vi "Read Settings File.vi"(8 "error in":errorcluster, 11 "Cluster in":T1 {"Gain Array"."Gain 17" format="%.2f"; "Gain Array"."Gain 16" format="%.2f"; "Gain Array"."Gain 15" format="%.2f"; "Gain Array"."Gain 14" format="%.2f"; "Gain Array"."Gain 13" format="%.2f"; "Gain Array"."Gain 12" format="%.2f"; "Gain Array"."Gain 11" format="%.2f"; "Gain Array"."Gain 10" format="%.2f"; "Gain Array"."Gain 9" format="%.2f"; "Gain Array"."Gain 8" format="%.2f"; "Gain Array"."Gain 7" format="%.2f"; "Gain Array"."Gain 6" format="%.2f"; "Gain Array"."Gain 5" format="%.2f"; "Gain Array"."Gain 4" format="%.2f"; "Gain Array"."Gain 3" format="%.2f"; "Gain Array"."Gain 2" format="%.2f"; "Gain Array"."Gain 1" format="%.2f"; "Gains"."Gain 6" format="%.2f"; "Gains"."Gain 5" format="%.2f"; "Gains"."Gain 4" format="%.2f"; "Gains"."Gain 3" format="%.2f"; "Gains"."Gain 2" format="%.2f"; "Gains"."Gain 1" format="%.2f"; "User Gains"."Gain 6" format="%.2f"; "User Gains"."Gain 5" format="%.2f"; "User Gains"."Gain 4" format="%.2f"; "User Gains"."Gain 3" format="%.2f"; "User Gains"."Gain 2" format="%.2f"; "User Gains"."Gain 1" format="%.2f"; "Channel Configuration List"."Channel Configuration Cluster 17"."Current Range" items=["1 <500m>"=0.5, "2 <1>"=1.0, "5 <2.5>"=2.5, "10 <5>"=5.0, "20 <10>"=10.0, "50 <25>"=25.0]; "Channel Configuration List"."Channel Configuration Cluster 17"."Voltage Range" items=["1.5 <0.75>"=0.75, "3 <1.5>"=1.5, "6 <3>"=3.0, "10 <5>"=5.0, "15 <7.5>"=7.5, "30 <15>"=15.0, "60 <30>"=30.0, "100 <50>"=50.0, "150 <75>"=75.0, "300 <150>"=150.0, "600 <300>"=300.0, "1000 <500>"=500.0]; "Channel Configuration List"."Channel Configuration Cluster 16"."Current Range" items=["1 <500m>"=0.5, "2 <1>"=1.0, "5 <2.5>"=2.5, "10 <5>"=5.0, "20 <10>"=10.0, "50 <25>"=25.0]; "Channel Configuration List"."Channel Configuration Cluster 16"."Voltage Range" items=["1.5 <0.75>"=0.75, "3 <1.5>"=1.5, "6 <3>"=3.0, "10 <5>"=5.0, "15 <7.5>"=7.5, "30 <15>"=15.0, "60 <30>"=30.0, "100 <50>"=50.0, "150 <75>"=75.0, "300 <150>"=150.0, "600 <300>"=300.0, "1000 <500>"=500.0]; "Channel Configuration List"."Channel Configuration Cluster 15"."Current Range" items=["1 <500m>"=0.5, "2 <1>"=1.0, "5 <2.5>"=2.5, "10 <5>"=5.0, "20 <10>"=10.0, "50 <25>"=25.0]; "Channel Configuration List"."Channel Configuration Cluster 15"."Voltage Range" items=["1.5 <0.75>"=0.75, "3 <1.5>"=1.5, "6 <3>"=3.0, "10 <5>"=5.0, "15 <7.5>"=7.5, "30 <15>"=15.0, "60 <30>"=30.0, "100 <50>"=50.0, "150 <75>"=75.0, "300 <150>"=150.0, "600 <300>"=300.0, "1000 <500>"=500.0]; "Channel Configuration List"."Channel Configuration Cluster 14"."Current Range" items=["1 <500m>"=0.5, "2 <1>"=1.0, "5 <2.5>"=2.5, "10 <5>"=5.0, "20 <10>"=10.0, "50 <25>"=25.0]; "Channel Configuration List"."Channel Configuration Cluster 14"."Voltage Range" items=["1.5 <0.75>"=0.75, "3 <1.5>"=1.5, "6 <3>"=3.0, "10 <5>"=5.0, "15 <7.5>"=7.5, "30 <15>"=15.0, "60 <30>"=30.0, "100 <50>"=50.0, "150 <75>"=75.0, "300 <150>"=150.0, "600 <300>"=300.0, "1000 <500>"=500.0]; "Channel Configuration List"."Channel Configuration Cluster 13"."Current Range" items=["1 <500m>"=0.5, "2 <1>"=1.0, "5 <2.5>"=2.5, "10 <5>"=5.0, "20 <10>"=10.0, "50 <25>"=25.0]; "Channel Configuration List"."Channel Configuration Cluster 13"."Voltage Range" items=["1.5 <0.75>"=0.75, "3 <1.5>"=1.5, "6 <3>"=3.0, "10 <5>"=5.0, "15 <7.5>"=7.5, "30 <15>"=15.0, "60 <30>"=30.0, "100 <50>"=50.0, "150 <75>"=75.0, "300 <150>"=150.0, "600 <300>"=300.0, "1000 <500>"=500.0]; "Channel Configuration List"."Channel Configuration Cluster 12"."Current Range" items=["1 <500m>"=0.5, "2 <1>"=1.0, "5 <2.5>"=2.5, "10 <5>"=5.0, "20 <10>"=10.0, "50 <25>"=25.0]; "Channel Configuration List"."Channel Configuration Cluster 12"."Voltage Range" items=["1.5 <0.75>"=0.75, "3 <1.5>"=1.5, "6 <3>"=3.0, "10 <5>"=5.0, "15 <7.5>"=7.5, "30 <15>"=15.0, "60 <30>"=30.0, "100 <50>"=50.0, "150 <75>"=75.0, "300 <150>"=150.0, "600 <300>"=300.0, "1000 <500>"=500.0]; "Channel Configuration List"."Channel Configuration Cluster 11"."Current Range" items=["1 <500m>"=0.5, "2 <1>"=1.0, "5 <2.5>"=2.5, "10 <5>"=5.0, "20 <10>"=10.0, "50 <25>"=25.0]; "Channel Configuration List"."Channel Configuration Cluster 11"."Voltage Range" items=["1.5 <0.75>"=0.75, "3 <1.5>"=1.5, "6 <3>"=3.0, "10 <5>"=5.0, "15 <7.5>"=7.5, "30 <15>"=15.0, "60 <30>"=30.0, "100 <50>"=50.0, "150 <75>"=75.0, "300 <150>"=150.0, "600 <300>"=300.0, "1000 <500>"=500.0]; "Channel Configuration List"."Channel Configuration Cluster 10"."Current Range" items=["1 <500m>"=0.5, "2 <1>"=1.0, "5 <2.5>"=2.5, "10 <5>"=5.0, "20 <10>"=10.0, "50 <25>"=25.0]; "Channel Configuration List"."Channel Configuration Cluster 10"."Voltage Range" items=["1.5 <0.75>"=0.75, "3 <1.5>"=1.5, "6 <3>"=3.0, "10 <5>"=5.0, "15 <7.5>"=7.5, "30 <15>"=15.0, "60 <30>"=30.0, "100 <50>"=50.0, "150 <75>"=75.0, "300 <150>"=150.0, "600 <300>"=300.0, "1000 <500>"=500.0]; "Channel Configuration List"."Channel Configuration Cluster 9"."Voltage Range" items=["1.5 <0.75>"=0.75, "3 <1.5>"=1.5, "6 <3>"=3.0, "10 <5>"=5.0, "15 <7.5>"=7.5, "30 <15>"=15.0, "60 <30>"=30.0, "100 <50>"=50.0, "150 <75>"=75.0, "300 <150>"=150.0, "600 <300>"=300.0, "1000 <500>"=500.0]; "Channel Configuration List"."Channel Configuration Cluster 9"."Current Range" items=["10m <5m>"=0.005, "20m <10m>"=0.01, "50m <25m>"=0.025, "100m <50m>"=0.05, "200m <100m>"=0.1, "500m <250m>"=0.25, "1 <500m>"=0.5, "2 <1>"=1.0, "5 <2.5>"=2.5]; "Channel Configuration List"."Channel Configuration Cluster 8"."Voltage Range" items=["1.5 <0.75>"=0.75, "3 <1.5>"=1.5, "6 <3>"=3.0, "10 <5>"=5.0, "15 <7.5>"=7.5, "30 <15>"=15.0, "60 <30>"=30.0, "100 <50>"=50.0, "150 <75>"=75.0, "300 <150>"=150.0, "600 <300>"=300.0, "1000 <500>"=500.0]; "Channel Configuration List"."Channel Configuration Cluster 8"."Current Range" items=["10m <5m>"=0.005, "20m <10m>"=0.01, "50m <25m>"=0.025, "100m <50m>"=0.05, "200m <100m>"=0.1, "500m <250m>"=0.25, "1 <500m>"=0.5, "2 <1>"=1.0, "5 <2.5>"=2.5]; "Channel Configuration List"."Channel Configuration Cluster 7"."Voltage Range" items=["1.5 <0.75>"=0.75, "3 <1.5>"=1.5, "6 <3>"=3.0, "10 <5>"=5.0, "15 <7.5>"=7.5, "30 <15>"=15.0, "60 <30>"=30.0, "100 <50>"=50.0, "150 <75>"=75.0, "300 <150>"=150.0, "600 <300>"=300.0, "1000 <500>"=500.0]; "Channel Configuration List"."Channel Configuration Cluster 7"."Current Range" items=["10m <5m>"=0.005, "20m <10m>"=0.01, "50m <25m>"=0.025, "100m <50m>"=0.05, "200m <100m>"=0.1, "500m <250m>"=0.25, "1 <500m>"=0.5, "2 <1>"=1.0, "5 <2.5>"=2.5]; "Channel Configuration List"."Channel Configuration Cluster 6"."Voltage Range" items=["1.5 <0.75>"=0.75, "3 <1.5>"=1.5, "6 <3>"=3.0, "10 <5>"=5.0, "15 <7.5>"=7.5, "30 <15>"=15.0, "60 <30>"=30.0, "100 <50>"=50.0, "150 <75>"=75.0, "300 <150>"=150.0, "600 <300>"=300.0, "1000 <500>"=500.0]; "Channel Configuration List"."Channel Configuration Cluster 6"."Current Range" items=["10m <5m>"=0.005, "20m <10m>"=0.01, "50m <25m>"=0.025, "100m <50m>"=0.05, "200m <100m>"=0.1, "500m <250m>"=0.25, "1 <500m>"=0.5, "2 <1>"=1.0, "5 <2.5>"=2.5]; "Channel Configuration List"."Channel Configuration Cluster 5"."Voltage Range" items=["1.5 <0.75>"=0.75, "3 <1.5>"=1.5, "6 <3>"=3.0, "10 <5>"=5.0, "15 <7.5>"=7.5, "30 <15>"=15.0, "60 <30>"=30.0, "100 <50>"=50.0, "150 <75>"=75.0, "300 <150>"=150.0, "600 <300>"=300.0, "1000 <500>"=500.0]; "Channel Configuration List"."Channel Configuration Cluster 5"."Current Range" items=["10m <5m>"=0.005, "20m <10m>"=0.01, "50m <25m>"=0.025, "100m <50m>"=0.05, "200m <100m>"=0.1, "500m <250m>"=0.25, "1 <500m>"=0.5, "2 <1>"=1.0, "5 <2.5>"=2.5]; "Channel Configuration List"."Channel Configuration Cluster 4"."Voltage Range" items=["1.5 <0.75>"=0.75, "3 <1.5>"=1.5, "6 <3>"=3.0, "10 <5>"=5.0, "15 <7.5>"=7.5, "30 <15>"=15.0, "60 <30>"=30.0, "100 <50>"=50.0, "150 <75>"=75.0, "300 <150>"=150.0, "600 <300>"=300.0, "1000 <500>"=500.0]; "Channel Configuration List"."Channel Configuration Cluster 4"."Current Range" items=["10m <5m>"=0.005, "20m <10m>"=0.01, "50m <25m>"=0.025, "100m <50m>"=0.05, "200m <100m>"=0.1, "500m <250m>"=0.25, "1 <500m>"=0.5, "2 <1>"=1.0, "5 <2.5>"=2.5]; "Channel Configuration List"."Channel Configuration Cluster 3"."Voltage Range" items=["1.5 <0.75>"=0.75, "3 <1.5>"=1.5, "6 <3>"=3.0, "10 <5>"=5.0, "15 <7.5>"=7.5, "30 <15>"=15.0, "60 <30>"=30.0, "100 <50>"=50.0, "150 <75>"=75.0, "300 <150>"=150.0, "600 <300>"=300.0, "1000 <500>"=500.0]; "Channel Configuration List"."Channel Configuration Cluster 3"."Current Range" items=["10m <5m>"=0.005, "20m <10m>"=0.01, "50m <25m>"=0.025, "100m <50m>"=0.05, "200m <100m>"=0.1, "500m <250m>"=0.25, "1 <500m>"=0.5, "2 <1>"=1.0, "5 <2.5>"=2.5]; "Channel Configuration List"."Channel Configuration Cluster 2"."Voltage Range" items=["1.5 <0.75>"=0.75, "3 <1.5>"=1.5, "6 <3>"=3.0, "10 <5>"=5.0, "15 <7.5>"=7.5, "30 <15>"=15.0, "60 <30>"=30.0, "100 <50>"=50.0, "150 <75>"=75.0, "300 <150>"=150.0, "600 <300>"=300.0, "1000 <500>"=500.0]; "Channel Configuration List"."Channel Configuration Cluster 2"."Current Range" items=["10m <5m>"=0.005, "20m <10m>"=0.01, "50m <25m>"=0.025, "100m <50m>"=0.05, "200m <100m>"=0.1, "500m <250m>"=0.25, "1 <500m>"=0.5, "2 <1>"=1.0, "5 <2.5>"=2.5]; "Channel Configuration List"."Channel Configuration Cluster"."Voltage Range" items=["1.5 <0.75>"=0.75, "3 <1.5>"=1.5, "6 <3>"=3.0, "10 <5>"=5.0, "15 <7.5>"=7.5, "30 <15>"=15.0, "60 <30>"=30.0, "100 <50>"=50.0, "150 <75>"=75.0, "300 <150>"=150.0, "600 <300>"=300.0, "1000 <500>"=500.0]; "Channel Configuration List"."Channel Configuration Cluster"."Current Range" items=["10m <5m>"=0.005, "20m <10m>"=0.01, "50m <25m>"=0.025, "100m <50m>"=0.05, "200m <100m>"=0.1, "500m <250m>"=0.25, "1 <500m>"=0.5, "2 <1>"=1.0, "5 <2.5>"=2.5]; "Settling Delay" min=0.0 format="%<%H:%M:%S>t"}) -> (0 "error out":errorcluster, 2 "status":bool, 3 "Cluster out":T1 {"Gain Array"."Gain 17" format="%.2f"; "Gain Array"."Gain 16" format="%.2f"; "Gain Array"."Gain 15" format="%.2f"; "Gain Array"."Gain 14" format="%.2f"; "Gain Array"."Gain 13" format="%.2f"; "Gain Array"."Gain 12" format="%.2f"; "Gain Array"."Gain 11" format="%.2f"; "Gain Array"."Gain 10" format="%.2f"; "Gain Array"."Gain 9" format="%.2f"; "Gain Array"."Gain 8" format="%.2f"; "Gain Array"."Gain 7" format="%.2f"; "Gain Array"."Gain 6" format="%.2f"; "Gain Array"."Gain 5" format="%.2f"; "Gain Array"."Gain 4" format="%.2f"; "Gain Array"."Gain 3" format="%.2f"; "Gain Array"."Gain 2" format="%.2f"; "Gain Array"."Gain 1" format="%.2f"; "Gains"."Gain 6" format="%.2f"; "Gains"."Gain 5" format="%.2f"; "Gains"."Gain 4" format="%.2f"; "Gains"."Gain 3" format="%.2f"; "Gains"."Gain 2" format="%.2f"; "Gains"."Gain 1" format="%.2f"; "User Gains"."Gain 6" format="%.2f"; "User Gains"."Gain 5" format="%.2f"; "User Gains"."Gain 4" format="%.2f"; "User Gains"."Gain 3" format="%.2f"; "User Gains"."Gain 2" format="%.2f"; "User Gains"."Gain 1" format="%.2f"; "Channel Configuration List"."Channel Configuration Cluster 17"."Current Range" items=["1 <500m>"=0.5, "2 <1>"=1.0, "5 <2.5>"=2.5, "10 <5>"=5.0, "20 <10>"=10.0, "50 <25>"=25.0]; "Channel Configuration List"."Channel Configuration Cluster 17"."Voltage Range" items=["1.5 <0.75>"=0.75, "3 <1.5>"=1.5, "6 <3>"=3.0, "10 <5>"=5.0, "15 <7.5>"=7.5, "30 <15>"=15.0, "60 <30>"=30.0, "100 <50>"=50.0, "150 <75>"=75.0, "300 <150>"=150.0, "600 <300>"=300.0, "1000 <500>"=500.0]; "Channel Configuration List"."Channel Configuration Cluster 16"."Current Range" items=["1 <500m>"=0.5, "2 <1>"=1.0, "5 <2.5>"=2.5, "10 <5>"=5.0, "20 <10>"=10.0, "50 <25>"=25.0]; "Channel Configuration List"."Channel Configuration Cluster 16"."Voltage Range" items=["1.5 <0.75>"=0.75, "3 <1.5>"=1.5, "6 <3>"=3.0, "10 <5>"=5.0, "15 <7.5>"=7.5, "30 <15>"=15.0, "60 <30>"=30.0, "100 <50>"=50.0, "150 <75>"=75.0, "300 <150>"=150.0, "600 <300>"=300.0, "1000 <500>"=500.0]; "Channel Configuration List"."Channel Configuration Cluster 15"."Current Range" items=["1 <500m>"=0.5, "2 <1>"=1.0, "5 <2.5>"=2.5, "10 <5>"=5.0, "20 <10>"=10.0, "50 <25>"=25.0]; "Channel Configuration List"."Channel Configuration Cluster 15"."Voltage Range" items=["1.5 <0.75>"=0.75, "3 <1.5>"=1.5, "6 <3>"=3.0, "10 <5>"=5.0, "15 <7.5>"=7.5, "30 <15>"=15.0, "60 <30>"=30.0, "100 <50>"=50.0, "150 <75>"=75.0, "300 <150>"=150.0, "600 <300>"=300.0, "1000 <500>"=500.0]; "Channel Configuration List"."Channel Configuration Cluster 14"."Current Range" items=["1 <500m>"=0.5, "2 <1>"=1.0, "5 <2.5>"=2.5, "10 <5>"=5.0, "20 <10>"=10.0, "50 <25>"=25.0]; "Channel Configuration List"."Channel Configuration Cluster 14"."Voltage Range" items=["1.5 <0.75>"=0.75, "3 <1.5>"=1.5, "6 <3>"=3.0, "10 <5>"=5.0, "15 <7.5>"=7.5, "30 <15>"=15.0, "60 <30>"=30.0, "100 <50>"=50.0, "150 <75>"=75.0, "300 <150>"=150.0, "600 <300>"=300.0, "1000 <500>"=500.0]; "Channel Configuration List"."Channel Configuration Cluster 13"."Current Range" items=["1 <500m>"=0.5, "2 <1>"=1.0, "5 <2.5>"=2.5, "10 <5>"=5.0, "20 <10>"=10.0, "50 <25>"=25.0]; "Channel Configuration List"."Channel Configuration Cluster 13"."Voltage Range" items=["1.5 <0.75>"=0.75, "3 <1.5>"=1.5, "6 <3>"=3.0, "10 <5>"=5.0, "15 <7.5>"=7.5, "30 <15>"=15.0, "60 <30>"=30.0, "100 <50>"=50.0, "150 <75>"=75.0, "300 <150>"=150.0, "600 <300>"=300.0, "1000 <500>"=500.0]; "Channel Configuration List"."Channel Configuration Cluster 12"."Current Range" items=["1 <500m>"=0.5, "2 <1>"=1.0, "5 <2.5>"=2.5, "10 <5>"=5.0, "20 <10>"=10.0, "50 <25>"=25.0]; "Channel Configuration List"."Channel Configuration Cluster 12"."Voltage Range" items=["1.5 <0.75>"=0.75, "3 <1.5>"=1.5, "6 <3>"=3.0, "10 <5>"=5.0, "15 <7.5>"=7.5, "30 <15>"=15.0, "60 <30>"=30.0, "100 <50>"=50.0, "150 <75>"=75.0, "300 <150>"=150.0, "600 <300>"=300.0, "1000 <500>"=500.0]; "Channel Configuration List"."Channel Configuration Cluster 11"."Current Range" items=["1 <500m>"=0.5, "2 <1>"=1.0, "5 <2.5>"=2.5, "10 <5>"=5.0, "20 <10>"=10.0, "50 <25>"=25.0]; "Channel Configuration List"."Channel Configuration Cluster 11"."Voltage Range" items=["1.5 <0.75>"=0.75, "3 <1.5>"=1.5, "6 <3>"=3.0, "10 <5>"=5.0, "15 <7.5>"=7.5, "30 <15>"=15.0, "60 <30>"=30.0, "100 <50>"=50.0, "150 <75>"=75.0, "300 <150>"=150.0, "600 <300>"=300.0, "1000 <500>"=500.0]; "Channel Configuration List"."Channel Configuration Cluster 10"."Current Range" items=["1 <500m>"=0.5, "2 <1>"=1.0, "5 <2.5>"=2.5, "10 <5>"=5.0, "20 <10>"=10.0, "50 <25>"=25.0]; "Channel Configuration List"."Channel Configuration Cluster 10"."Voltage Range" items=["1.5 <0.75>"=0.75, "3 <1.5>"=1.5, "6 <3>"=3.0, "10 <5>"=5.0, "15 <7.5>"=7.5, "30 <15>"=15.0, "60 <30>"=30.0, "100 <50>"=50.0, "150 <75>"=75.0, "300 <150>"=150.0, "600 <300>"=300.0, "1000 <500>"=500.0]; "Channel Configuration List"."Channel Configuration Cluster 9"."Voltage Range" items=["1.5 <0.75>"=0.75, "3 <1.5>"=1.5, "6 <3>"=3.0, "10 <5>"=5.0, "15 <7.5>"=7.5, "30 <15>"=15.0, "60 <30>"=30.0, "100 <50>"=50.0, "150 <75>"=75.0, "300 <150>"=150.0, "600 <300>"=300.0, "1000 <500>"=500.0]; "Channel Configuration List"."Channel Configuration Cluster 9"."Current Range" items=["10m <5m>"=0.005, "20m <10m>"=0.01, "50m <25m>"=0.025, "100m <50m>"=0.05, "200m <100m>"=0.1, "500m <250m>"=0.25, "1 <500m>"=0.5, "2 <1>"=1.0, "5 <2.5>"=2.5]; "Channel Configuration List"."Channel Configuration Cluster 8"."Voltage Range" items=["1.5 <0.75>"=0.75, "3 <1.5>"=1.5, "6 <3>"=3.0, "10 <5>"=5.0, "15 <7.5>"=7.5, "30 <15>"=15.0, "60 <30>"=30.0, "100 <50>"=50.0, "150 <75>"=75.0, "300 <150>"=150.0, "600 <300>"=300.0, "1000 <500>"=500.0]; "Channel Configuration List"."Channel Configuration Cluster 8"."Current Range" items=["10m <5m>"=0.005, "20m <10m>"=0.01, "50m <25m>"=0.025, "100m <50m>"=0.05, "200m <100m>"=0.1, "500m <250m>"=0.25, "1 <500m>"=0.5, "2 <1>"=1.0, "5 <2.5>"=2.5]; "Channel Configuration List"."Channel Configuration Cluster 7"."Voltage Range" items=["1.5 <0.75>"=0.75, "3 <1.5>"=1.5, "6 <3>"=3.0, "10 <5>"=5.0, "15 <7.5>"=7.5, "30 <15>"=15.0, "60 <30>"=30.0, "100 <50>"=50.0, "150 <75>"=75.0, "300 <150>"=150.0, "600 <300>"=300.0, "1000 <500>"=500.0]; "Channel Configuration List"."Channel Configuration Cluster 7"."Current Range" items=["10m <5m>"=0.005, "20m <10m>"=0.01, "50m <25m>"=0.025, "100m <50m>"=0.05, "200m <100m>"=0.1, "500m <250m>"=0.25, "1 <500m>"=0.5, "2 <1>"=1.0, "5 <2.5>"=2.5]; "Channel Configuration List"."Channel Configuration Cluster 6"."Voltage Range" items=["1.5 <0.75>"=0.75, "3 <1.5>"=1.5, "6 <3>"=3.0, "10 <5>"=5.0, "15 <7.5>"=7.5, "30 <15>"=15.0, "60 <30>"=30.0, "100 <50>"=50.0, "150 <75>"=75.0, "300 <150>"=150.0, "600 <300>"=300.0, "1000 <500>"=500.0]; "Channel Configuration List"."Channel Configuration Cluster 6"."Current Range" items=["10m <5m>"=0.005, "20m <10m>"=0.01, "50m <25m>"=0.025, "100m <50m>"=0.05, "200m <100m>"=0.1, "500m <250m>"=0.25, "1 <500m>"=0.5, "2 <1>"=1.0, "5 <2.5>"=2.5]; "Channel Configuration List"."Channel Configuration Cluster 5"."Voltage Range" items=["1.5 <0.75>"=0.75, "3 <1.5>"=1.5, "6 <3>"=3.0, "10 <5>"=5.0, "15 <7.5>"=7.5, "30 <15>"=15.0, "60 <30>"=30.0, "100 <50>"=50.0, "150 <75>"=75.0, "300 <150>"=150.0, "600 <300>"=300.0, "1000 <500>"=500.0]; "Channel Configuration List"."Channel Configuration Cluster 5"."Current Range" items=["10m <5m>"=0.005, "20m <10m>"=0.01, "50m <25m>"=0.025, "100m <50m>"=0.05, "200m <100m>"=0.1, "500m <250m>"=0.25, "1 <500m>"=0.5, "2 <1>"=1.0, "5 <2.5>"=2.5]; "Channel Configuration List"."Channel Configuration Cluster 4"."Voltage Range" items=["1.5 <0.75>"=0.75, "3 <1.5>"=1.5, "6 <3>"=3.0, "10 <5>"=5.0, "15 <7.5>"=7.5, "30 <15>"=15.0, "60 <30>"=30.0, "100 <50>"=50.0, "150 <75>"=75.0, "300 <150>"=150.0, "600 <300>"=300.0, "1000 <500>"=500.0]; "Channel Configuration List"."Channel Configuration Cluster 4"."Current Range" items=["10m <5m>"=0.005, "20m <10m>"=0.01, "50m <25m>"=0.025, "100m <50m>"=0.05, "200m <100m>"=0.1, "500m <250m>"=0.25, "1 <500m>"=0.5, "2 <1>"=1.0, "5 <2.5>"=2.5]; "Channel Configuration List"."Channel Configuration Cluster 3"."Voltage Range" items=["1.5 <0.75>"=0.75, "3 <1.5>"=1.5, "6 <3>"=3.0, "10 <5>"=5.0, "15 <7.5>"=7.5, "30 <15>"=15.0, "60 <30>"=30.0, "100 <50>"=50.0, "150 <75>"=75.0, "300 <150>"=150.0, "600 <300>"=300.0, "1000 <500>"=500.0]; "Channel Configuration List"."Channel Configuration Cluster 3"."Current Range" items=["10m <5m>"=0.005, "20m <10m>"=0.01, "50m <25m>"=0.025, "100m <50m>"=0.05, "200m <100m>"=0.1, "500m <250m>"=0.25, "1 <500m>"=0.5, "2 <1>"=1.0, "5 <2.5>"=2.5]; "Channel Configuration List"."Channel Configuration Cluster 2"."Voltage Range" items=["1.5 <0.75>"=0.75, "3 <1.5>"=1.5, "6 <3>"=3.0, "10 <5>"=5.0, "15 <7.5>"=7.5, "30 <15>"=15.0, "60 <30>"=30.0, "100 <50>"=50.0, "150 <75>"=75.0, "300 <150>"=150.0, "600 <300>"=300.0, "1000 <500>"=500.0]; "Channel Configuration List"."Channel Configuration Cluster 2"."Current Range" items=["10m <5m>"=0.005, "20m <10m>"=0.01, "50m <25m>"=0.025, "100m <50m>"=0.05, "200m <100m>"=0.1, "500m <250m>"=0.25, "1 <500m>"=0.5, "2 <1>"=1.0, "5 <2.5>"=2.5]; "Channel Configuration List"."Channel Configuration Cluster"."Voltage Range" items=["1.5 <0.75>"=0.75, "3 <1.5>"=1.5, "6 <3>"=3.0, "10 <5>"=5.0, "15 <7.5>"=7.5, "30 <15>"=15.0, "60 <30>"=30.0, "100 <50>"=50.0, "150 <75>"=75.0, "300 <150>"=150.0, "600 <300>"=300.0, "1000 <500>"=500.0]; "Channel Configuration List"."Channel Configuration Cluster"."Current Range" items=["10m <5m>"=0.005, "20m <10m>"=0.01, "50m <25m>"=0.025, "100m <50m>"=0.05, "200m <100m>"=0.1, "500m <250m>"=0.25, "1 <500m>"=0.5, "2 <1>"=1.0, "5 <2.5>"=2.5]; "Settling Delay" min=0.0 format="%<%H:%M:%S>t"})   [LabVIEW 2021]
uses:
  Controls/Settings Control.ctl
  Controls/Channel Configuration List.ctl
  Controls/Channel Configuration Cluster.ctl
  Controls/Channel Configuration Cluster High Current.ctl
  Controls/Gain Averages.ctl
  Controls/Gain Array.ctl
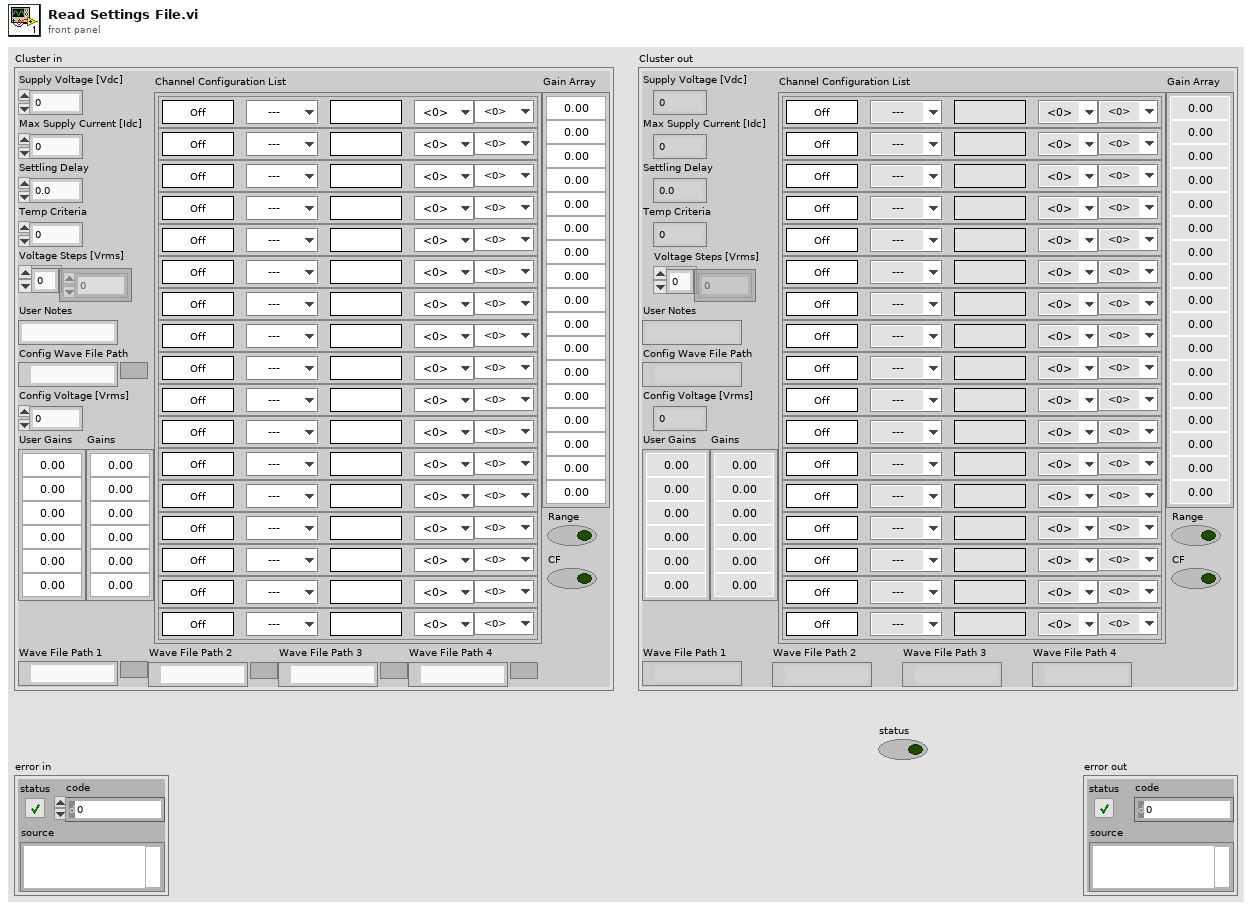
[diagram p1: front panel]
types:
  T1 = typedef "Settings Control.ctl" = cluster{"Supply Voltage [Vdc]":sgl, "Max Supply Current [Idc]":sgl, "Settling Delay":dbl, "Temp Criteria":sgl, "Voltage Steps [Vrms]":sgl[], "User Notes":string, "Config Wave File Path":path, "Config Voltage [Vrms]":sgl, "Channel Configuration List":T2, "User Gains":T5, "Gains":T5, "Gain Array":T6, "Wave File Path 1":path, "Wave File Path 2":path, "Wave File Path 3":path, "Wave File Path 4":path, "Range":bool, "CF":bool}
  T2 = typedef "Channel Configuration List.ctl" = cluster{"Channel Configuration Cluster":T3, "Channel Configuration Cluster 2":T3, "Channel Configuration Cluster 3":T3, "Channel Configuration Cluster 4":T3, "Channel Configuration Cluster 5":T3, "Channel Configuration Cluster 6":T3, "Channel Configuration Cluster 7":T3, "Channel Configuration Cluster 8":T3, "Channel Configuration Cluster 9":T3, "Channel Configuration Cluster 10":T4, "Channel Configuration Cluster 11":T4, "Channel Configuration Cluster 12":T4, "Channel Configuration Cluster 13":T4, "Channel Configuration Cluster 14":T4, "Channel Configuration Cluster 15":T4, "Channel Configuration Cluster 16":T4, "Channel Configuration Cluster 17":T4}
  T3 = typedef "Channel Configuration Cluster.ctl" = cluster{"Input":enum16{"---", "1", "1 AVG", "2", "2 AVG", "3", "3 AVG", "4", "4 AVG"}, "Enable":bool, "User Notes":string, "Voltage Range":dbl, "Current Range":dbl}
  T4 = typedef "Channel Configuration Cluster High Current.ctl" = cluster{"Input":enum16{"---", "1", "1 AVG", "2", "2 AVG", "3", "3 AVG", "4", "4 AVG"}, "Enable":bool, "User Notes":string, "Voltage Range":dbl, "Current Range":dbl}
  T5 = typedef "Gain Averages.ctl" = cluster{"Gain 1":dbl, "Gain 2":dbl, "Gain 3":dbl, "Gain 4":dbl, "Gain 5":dbl, "Gain 6":dbl}
  T6 = typedef "Gain Array.ctl" = cluster{"Gain 1":dbl, "Gain 2":dbl, "Gain 3":dbl, "Gain 4":dbl, "Gain 5":dbl, "Gain 6":dbl, "Gain 7":dbl, "Gain 8":dbl, "Gain 9":dbl, "Gain 10":dbl, "Gain 11":dbl, "Gain 12":dbl, "Gain 13":dbl, "Gain 14":dbl, "Gain 15":dbl, "Gain 16":dbl, "Gain 17":dbl}
  T7 = cluster{"Supply Voltage [Vdc]":dbl, "Max Supply Current [Idc]":dbl, "Settling Delay":dbl, "Temp Criteria":dbl, "Voltage Steps [Vrms]":dbl[], "User Notes":string, "Config Wave File Path":path, "Config Voltage [Vrms]":dbl, "Channel Configuration List":T2, "User Gains":T5, "Gains":T5, "Gain Array":T6, "Wave File Path 1":path, "Wave File Path 2":path, "Wave File Path 3":path, "Wave File Path 4":path}
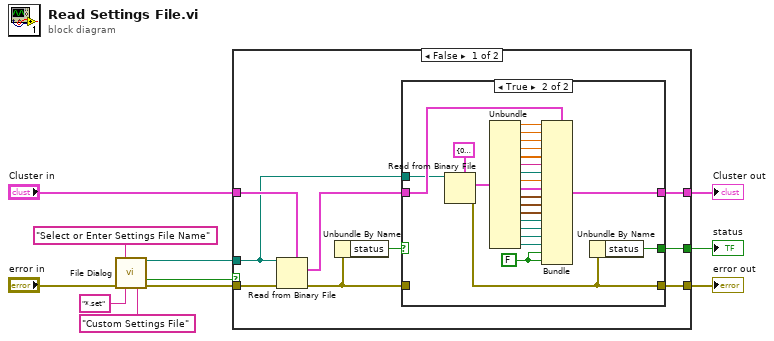
[diagram p0: block diagram]
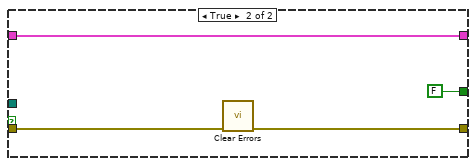
[diagram p3: hidden frame]
diagram:
  n1 = call "File Dialog"("prompt"="Select or Enter Settings File Name", "error in"="error in", "pattern (all files)"="*.set", "pattern label"="Custom Settings File") -> ("selected path"=w9:path, "cancelled"=w11:bool, "error out"=w10:errorcluster)  [unwired: 8 in, 1 out]
  n2 = case shown="False" w11 {
    tunnel: [w15 w50] -> w5
    tunnel: w9 -> [w12 _]
    tunnel: w10 -> [w20 w51]
    tunnel: [w13 w49] -> w1
    tunnel: "Cluster in" -> [w19 w49]
    tunnel: [w16 FALSE ("status")] -> w3
    frame False {
      n3 = Read from Binary File(5:w19, 8:w20, 11:w12) -> (0:w17:errorcluster, 2:w14:T1)  [unwired: 3 in, 2 out]
      n4 = Unbundle By Name(w17) -> ("status"=w18:bool)
      n5 = case shown="True" w18 {
        selector: w18 -> [w22 _]
        tunnel: [w23 w27] -> w15
        tunnel: w17 -> [w23 _]
        tunnel: [w22 w26] -> w16
        tunnel: [w21 w25] -> w13
        tunnel: w14 -> [w21 w28]
        tunnel: w12 -> [_ w24]
        frame False {
        }
        frame True {
          w31 = FALSE ("CF")
          n6 = Read from Binary File(5:T7 {"Supply Voltage [Vdc]"=0.0, "Max Supply Current [Idc]"=0.0, "Settling Delay"=0.0, "Temp Criteria"=0.0, "Voltage Steps [Vrms]"=[], "User Notes"="", "Config Wave File Path"=path "", "Config Voltage [Vrms]"=0.0, "Channel Configuration List"={"Channel Configuration Cluster"={"Input"=enum."---", "Enable"=FALSE, "User Notes"="", "Voltage Range"=0.0, "Current Range"=0.0}, "Channel Configuration Cluster 2"={"Input"=enum."---", "Enable"=FALSE, "User Notes"="", "Voltage Range"=0.0, "Current Range"=0.0}, "Channel Configuration Cluster 3"={"Input"=enum."---", "Enable"=FALSE, "User Notes"="", "Voltage Range"=0.0, "Current Range"=0.0}, "Channel Configuration Cluster 4"={"Input"=enum."---", "Enable"=FALSE, "User Notes"="", "Voltage Range"=0.0, "Current Range"=0.0}, "Channel Configuration Cluster 5"={"Input"=enum."---", "Enable"=FALSE, "User Notes"="", "Voltage Range"=0.0, "Current Range"=0.0}, "Channel Configuration Cluster 6"={"Input"=enum."---", "Enable"=FALSE, "User Notes"="", "Voltage Range"=0.0, "Current Range"=0.0}, "Channel Configuration Cluster 7"={"Input"=enum."---", "Enable"=FALSE, "User Notes"="", "Voltage Range"=0.0, "Current Range"=0.0}, "Channel Configuration Cluster 8"={"Input"=enum."---", "Enable"=FALSE, "User Notes"="", "Voltage Range"=0.0, "Current Range"=0.0}, "Channel Configuration Cluster 9"={"Input"=enum."---", "Enable"=FALSE, "User Notes"="", "Voltage Range"=0.0, "Current Range"=0.0}, "Channel Configuration Cluster 10"={"Input"=enum."---", "Enable"=FALSE, "User Notes"="", "Voltage Range"=0.0, "Current Range"=0.0}, "Channel Configuration Cluster 11"={"Input"=enum."---", "Enable"=FALSE, "User Notes"="", "Voltage Range"=0.0, "Current Range"=0.0}, "Channel Configuration Cluster 12"={"Input"=enum."---", "Enable"=FALSE, "User Notes"="", "Voltage Range"=0.0, "Current Range"=0.0}, "Channel Configuration Cluster 13"={"Input"=enum."---", "Enable"=FALSE, "User Notes"="", "Voltage Range"=0.0, "Current Range"=0.0}, "Channel Configuration Cluster 14"={"Input"=enum."---", "Enable"=FALSE, "User Notes"="", "Voltage Range"=0.0, "Current Range"=0.0}, "Channel Configuration Cluster 15"={"Input"=enum."---", "Enable"=FALSE, "User Notes"="", "Voltage Range"=0.0, "Current Range"=0.0}, "Channel Configuration Cluster 16"={"Input"=enum."---", "Enable"=FALSE, "User Notes"="", "Voltage Range"=0.0, "Current Range"=0.0}, "Channel Configuration Cluster 17"={"Input"=enum."---", "Enable"=FALSE, "User Notes"="", "Voltage Range"=0.0, "Current Range"=0.0}}, "User Gains"={"Gain 1"=0.0, "Gain 2"=0.0, "Gain 3"=0.0, "Gain 4"=0.0, "Gain 5"=0.0, "Gain 6"=0.0}, "Gains"={"Gain 1"=0.0, "Gain 2"=0.0, "Gain 3"=0.0, "Gain 4"=0.0, "Gain 5"=0.0, "Gain 6"=0.0}, "Gain Array"={"Gain 1"=0.0, "Gain 2"=0.0, "Gain 3"=0.0, "Gain 4"=0.0, "Gain 5"=0.0, "Gain 6"=0.0, "Gain 7"=0.0, "Gain 8"=0.0, "Gain 9"=0.0, "Gain 10"=0.0, "Gain 11"=0.0, "Gain 12"=0.0, "Gain 13"=0.0, "Gain 14"=0.0, "Gain 15"=0.0, "Gain 16"=0.0, "Gain 17"=0.0}, "Wave File Path 1"=path "", "Wave File Path 2"=path "", "Wave File Path 3"=path "", "Wave File Path 4"=path ""} ("Cluster out"), 11:w24) -> (0:w27:errorcluster, 2:w30:T7)  [unwired: 4 in, 2 out]
          n7 = Unbundle(w30) -> ("Supply Voltage [Vdc]"=w47:dbl, "Max Supply Current [Idc]"=w46:dbl, "Settling Delay"=w45:dbl, "Temp Criteria"=w44:dbl, "Voltage Steps [Vrms]"=w32:dbl[], "User Notes"=w33:string, "Config Wave File Path"=w34:path, "Config Voltage [Vrms]"=w35:dbl, "Channel Configuration List"=w36:T2, "User Gains"=w37:T5, "Gains"=w38:T5, "Gain Array"=w39:T6, "Wave File Path 1"=w40:path, "Wave File Path 2"=w41:path, "Wave File Path 3"=w42:path, "Wave File Path 4"=w43:path)
          n8 = Bundle(cluster=w28, "Supply Voltage [Vdc]"=w47, "Max Supply Current [Idc]"=w46, "Settling Delay"=w45, "Temp Criteria"=w44, "Voltage Steps [Vrms]"=w32, "User Notes"=w33, "Config Wave File Path"=w34, "Config Voltage [Vrms]"=w35, "Channel Configuration List"=w36, "User Gains"=w37, "Gains"=w38, "Gain Array"=w39, "Wave File Path 1"=w40, "Wave File Path 2"=w41, "Wave File Path 3"=w42, "Wave File Path 4"=w43, "Range"=w31, "CF"=w31) -> (w25:T1)
          n9 = Unbundle By Name(w27) -> ("status"=w26:bool)
        }
      }
    }
    frame True {
      n10 = call <vilib>:"Clear Errors.vi"("error in (no error)"=w51) -> ("error out"=w50:errorcluster)  [unwired: 5 in, 1 out]
    }
  }
  "error out" <- w5
  "status" <- w3
  "Cluster out" <- w1
